vi "REPORT_DATES_rows_style_pdf.vi"(11 "REPORT_GEAR_all_info":T1) -> (3 "Row  [ ]":T3)   [LabVIEW 2019]
uses:
  <vilib>/Exaprom PDF/Controls/Table Controls/Table Appearance and Font Row [ ].ctl
  <vilib>/Exaprom PDF/Controls/Table Controls/One Row Appearance.ctl
  <vilib>/Exaprom PDF/Controls/Table Controls/Row from to.ctl
  <vilib>/Exaprom PDF/Controls/Table Controls/Cell, Alignment, LS and Font - hide Vmerge.ctl
  <vilib>/Exaprom PDF/Controls/Table Controls/Cell Type, Alignment and LS.ctl
  <vilib>/Exaprom PDF/Controls/Table Controls/Cell Alignment 20px.ctl
  <vilib>/Exaprom PDF/Controls/Table Controls/Text vertical arrangement.ctl
  <vilib>/Exaprom PDF/Controls/Text Controls/Line spacing.ctl
  <vilib>/Exaprom PDF/Controls/Table Controls/Cell Appearance.ctl
  <vilib>/Exaprom PDF/Controls/Table Controls/Cell Border 20 px.ctl
  <vilib>/Exaprom PDF/Controls/Table Controls/Merge Horizontal.ctl
  <vilib>/Exaprom PDF/Controls/Table Controls/Merge Vertical.ctl
  <vilib>/Exaprom PDF/Controls/Font Controls/Font complete cluster.ctl
  <vilib>/Exaprom PDF/Controls/Font Controls/Font size.ctl
  <vilib>/Exaprom PDF/Controls/Font Controls/Font color.ctl
  <vilib>/Exaprom PDF/Controls/Font Controls/Type and encoding.ctl
  <vilib>/Exaprom PDF/Controls/Text Controls/Unicode/Type and run direction.ctl
  typedef/REPORT_DATES_all_info.ctl
  typedef/REPORT_DATES_statuses.ctl
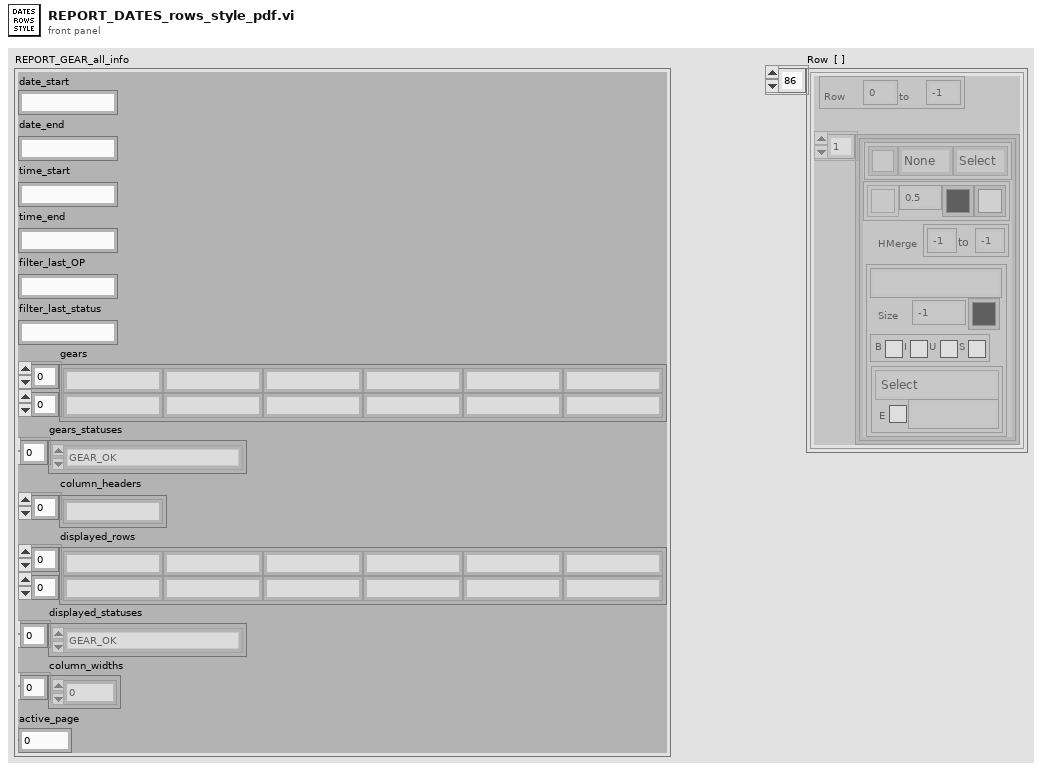
[diagram p1: front panel]
types:
  T1 = typedef "REPORT_DATES_all_info.ctl" = cluster{"date_start":string, "date_end":string, "time_start":string, "time_end":string, "filter_last_OP":string, "filter_last_status":string, "gears":string[][], "gears_statuses":T2[], "column_headers":string[], "displayed_rows":string[][], "displayed_statuses":T2[], "column_widths":i16[], "active_page":i32}
  T2 = typedef "REPORT_DATES_statuses.ctl" = enum16{"GEAR_OK", "GEAR_NOK", "GEAR_interrupted", "GEAR_in_operation", "GEAR_unexpected"}
  T3 = typedef "Table Appearance and Font Row [ ].ctl" = T4[]
  T4 = typedef "One Row Appearance.ctl" = cluster{"Row":T5, "Cell [ ]":T6[]}
  T5 = typedef "Row from to.ctl" = cluster{"From #":i16, "to #":i16}
  T6 = typedef "Cell, Alignment, LS and Font - hide Vmerge.ctl" = cluster{"Text":T7, "Cell Appearance":T11, "HMerge":T13, "VMerge":T14, "Font":T15}
  T7 = typedef "Cell Type, Alignment and LS.ctl" = cluster{"Cell Alignment":T8, "Text rotation":T9, "Line spacing":T10}
  T8 = typedef "Cell Alignment 20px.ctl" = u16
  T9 = typedef "Text vertical arrangement.ctl" = enum16{"None", "Clockwise", "Counterclockwise"}
  T10 = typedef "Line spacing.ctl" = enum16{"Select", "1.0", "1.5", "2.0"}
  T11 = typedef "Cell Appearance.ctl" = cluster{"Border":T12, "Thickness":sgl, "Color":u32, "BG":u32}
  T12 = typedef "Cell Border 20 px.ctl" = u16
  T13 = typedef "Merge Horizontal.ctl" = cluster{"From":i8, "to":i8}
  T14 = typedef "Merge Vertical.ctl" = cluster{"From":i8, "to":i8}
  T15 = typedef "Font complete cluster.ctl" = cluster{"Name":string, "Size":T16, "Color":T17, "Style":cluster{"Bold":bool, "Italic":bool, "Underline":bool, "Strikeout":bool}, "Type":T18}
  T16 = typedef "Font size.ctl" = sgl
  T17 = typedef "Font color.ctl" = u32
  T18 = typedef "Type and encoding.ctl" = cluster{"Type&direction":T19, "Embedded":bool, "Encoding":string}
  T19 = typedef "Type and run direction.ctl" = enum16{"Select", "ASCII", "UTF-16", "UTF-16 (default)", "UTF-16 (LTR)", "UTF-16 (RTL)"}
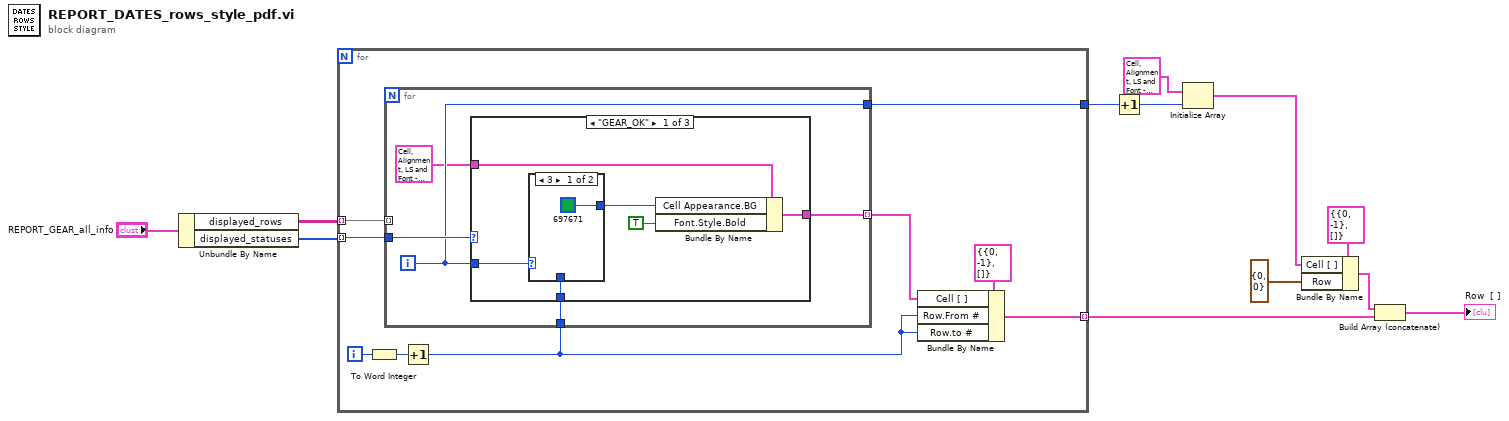
[diagram p0: block diagram]
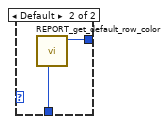
[diagram p2: hidden frame]
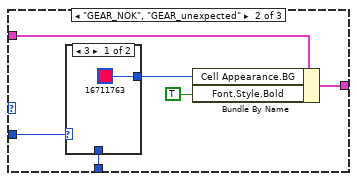
[diagram p3: hidden frame]
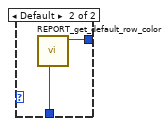
[diagram p4: hidden frame]
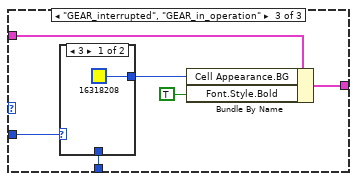
[diagram p5: hidden frame]
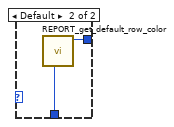
[diagram p6: hidden frame]
diagram:
  n1 = Unbundle By Name("REPORT_GEAR_all_info") -> ("displayed_rows"=w11:string[][], "displayed_statuses"=w10:T2[])
  n2 = for {
    tunnel: w11 -> [w17] mode=indexing
    tunnel: w10 -> [w16] mode=indexing
    tunnel: [w20] -> w8 mode=indexing
    tunnel: [w13] -> w2
    i -> [w19]
    n3 = To Word Integer(number=w19) -> (16bit integer=w18:i16)
    n4 = Increment(x=w18) -> (x+1=w14:i16)
    n5 = for {
      tunnel: w17 -> [_] mode=indexing
      tunnel: w16 -> [w26]
      tunnel: [w25] -> w15 mode=indexing
      tunnel: w14 -> [w24]
      tunnel: [w23] -> w13
      i -> [w23]
      n6 = case shown="\"GEAR_OK\"" w26 {
        tunnel: T6 {"Text"={"Cell Alignment"=0, "Text rotation"=enum."None", "Line spacing"=enum."Select"}, "Cell Appearance"={"Border"=5, "Thickness"=0.5, "Color"=0, "BG"=16448250}, "HMerge"={"From"=-1, "to"=-1}, "VMerge"={"From"=-1, "to"=-1}, "Font"={"Name"="Consolas", "Size"=10.0, "Color"=0, "Style"={"Bold"=FALSE, "Italic"=FALSE, "Underline"=FALSE, "Strikeout"=FALSE}, "Type"={"Type&direction"=enum."ASCII", "Embedded"=FALSE, "Encoding"="CP855"}}} ("Cell, Alignment, LS and Font") -> [w32 w39 w48]
        tunnel: [w29 w38 w47] -> w25
        tunnel: w23 -> [w28 w37 w46]
        tunnel: w24 -> [w27 w36 w45]
        frame "GEAR_OK" {
          n7 = case shown="3" w28 {
            tunnel: [u32 697671 w35] -> w30
            tunnel: w27 -> [_ w34]
            frame 3 {
            }
            frame Default {
              n8 = call "REPORT_get_default_row_color.vi"("row"=w34) -> ("color"=w35:u32)  [unwired: 10 in]
            }
          }
          n9 = Bundle By Name(cluster=w32, "Cell Appearance.BG"=w30, "Font.Style.Bold"=TRUE ("Active Cell:Cell Font:Bold")) -> (w29:T6)
        }
        frame "GEAR_NOK", "GEAR_unexpected" {
          n10 = case shown="3" w37 {
            tunnel: [u32 16711763 w44] -> w40
            tunnel: w36 -> [_ w43]
            frame 3 {
            }
            frame Default {
              n11 = call "REPORT_get_default_row_color.vi"("row"=w43) -> ("color"=w44:u32)  [unwired: 10 in]
            }
          }
          n12 = Bundle By Name(cluster=w39, "Cell Appearance.BG"=w40, "Font.Style.Bold"=TRUE ("Active Cell:Cell Font:Bold")) -> (w38:T6)
        }
        frame "GEAR_interrupted", "GEAR_in_operation" {
          n13 = case shown="3" w46 {
            tunnel: [u32 16318208 w53] -> w49
            tunnel: w45 -> [_ w52]
            frame 3 {
            }
            frame Default {
              n14 = call "REPORT_get_default_row_color.vi"("row"=w52) -> ("color"=w53:u32)  [unwired: 10 in]
            }
          }
          n15 = Bundle By Name(cluster=w48, "Cell Appearance.BG"=w49, "Font.Style.Bold"=TRUE ("Active Cell:Cell Font:Bold")) -> (w47:T6)
        }
      }
    }
    n16 = Bundle By Name(cluster=T4 {"Row"={"From #"=0, "to #"=-1}, "Cell [ ]"=[]} ("Row Appearance and Font  [ ]"), "Cell [ ]"=w15, "Row.From #"=w14, "Row.to #"=w14) -> (w20:T4)
  }
  n17 = Increment(x=w2) -> (x+1=w1:i32)
  n18 = Initialize Array(T6 {"Text"={"Cell Alignment"=0, "Text rotation"=enum."None", "Line spacing"=enum."Select"}, "Cell Appearance"={"Border"=5, "Thickness"=1.5, "Color"=16777228, "BG"=16448250}, "HMerge"={"From"=-1, "to"=-1}, "VMerge"={"From"=-1, "to"=-1}, "Font"={"Name"="Consolas", "Size"=10.0, "Color"=16777228, "Style"={"Bold"=TRUE, "Italic"=FALSE, "Underline"=FALSE, "Strikeout"=FALSE}, "Type"={"Type&direction"=enum."ASCII", "Embedded"=FALSE, "Encoding"="CP855"}}} ("Cell, Alignment, LS and Font"), w1) -> (w4:T6[])
  n19 = Bundle By Name(cluster=T4 {"Row"={"From #"=0, "to #"=-1}, "Cell [ ]"=[]} ("Row Appearance and Font  [ ]"), "Cell [ ]"=w4, "Row"=T5 {"From #"=0, "to #"=0}) -> (w6:T4)
  n20 = Build Array (concatenate)(w6, w8) -> (→"Row  [ ]":T4[])
